vi "DPT Global Test Variables.vi"() -> ()   [LabVIEW 2016, in "File Setup.lvlib"]
uses:
  File Setup.lvlib
  Type Definition/DPT Global Type.ctl
panel:
  in  "34970 RDB Chan":string="101"
  in  "34970 ChTemp Chan":string="113"
  in  "34970 RH Chan":string="112"
  in  "34970 Weight Chan":string="111"
  in  "34970 Label List":string[](array[string])=["RDB F", "Room Ambient(F)", "TC 103", "TC 104", "TC 105", "TC 106", "TC 107", "TC 108", "TC 109", "TC 110"]
  in  "34970 TC Chan List":string="101,102,103,104,105,106,107,108,109,110"
  in  "Corrected Weight Header":string="Corrected Weight"
  in  "Raw Weight Header":string="Raw Weight"
  in  "Weight Header":string="Weight"
  in  "TT3 Header":string="TIME TO 3% RMC:"
  in  "TT4 Header":string="TIME TO 4% RMC:"
  in  "TT5 Header":string="TIME TO 5% RMC:"
  in  "Gas Press Header":string="Gas Pressure"
  in  "Gas Temp Header":string="Gas Temperature"
  in  "Gas Vol Header":string="Gas Feedback"
  in  "Bar. Pressure Header":string="Barometric Pressure"
  in  "WattHour Header":string="Wp:Sigma"
  in  "RMC Header":string="RMC"
  in  "Time Header":string="Time"
  in  "Frequency Label":string="FREQUENCY (Hz):"
  in  "Date Label":string="DATE:"
  in  "IL2 Header":string="Irms:Element 2"
  in  "Dryer On Min Current":dbl=1.0
  in  "IL1 Header":string="Irms:Element 1"
  in  "RH Header":string="Chamber RH"
  in  "Tambient Header":string="Room Ambient(F)"
  in  "VL2 Header":string="Urms:Element 2"
  in  "VL1 Header":string="Urms:Element 1"
  in  "Header Search Key2":string="Date"
  in  "Header Search Key1":string="Time"
  in  "Globals for Dryer Performance Test":T1={"Test Setup"={"RH Resistor"=100.0, "Temp Cal"=72.0, "Temp Coeff"=-0.0234, "Power On Threshold"=50.0, "MA Filter Size"=60, "Weight Offset"=0.0, "Temp Resistor"=100.0, "Gas Enabled"=FALSE, "Gas P. Resistor"=250.0, "Scale Com"=1.0, "W. Samps"=5, "Temp4mA Val"=32.0, "Temp20mA Val"=212.0, "RH4mA Val"=0.0, "RH20mA Val"=100.0, "GPres4mA Val"=0.0, "Gpres20mA Val"=50.0, "Smoothing"=FALSE, "CDAQ"=FALSE, "34970"=FALSE, "34980"=FALSE, "RH-IP"="192.168.1.161", "RH-IP2"="192.168.1.41", "RH-IP3"="192.168.1.42", "CompVolume"=0.0, "T45_Coeff."=0.0}, "Agilent Setup"={"Scale Channel"="3009", "TC Channels"="1001:1040,2001:2040", "VDC Discrete Channels"="3001:3008", "RH Chan"="3010", "Temp Chan"="3011", "Tscale Channel"="1003", "RDB Channel"="1001", "Gas Temperature"="1019", "Gas Pressure"="1020", "Barometric Pressure"="1040", "Gas Feedback Chan"="3012"}, "Directories"={"Work File Directory"=path "c:/Work", "Save File Directory"=path "c:/Data", "Library Directory"=path "c:/Data", "Data Backup Directory"=path "c:/Data", "Data Backup Dir Fail"=path "c:/Data", "Lab Directory"=path "c:/Data"}, "Test Information"={"Model:"="", "Temperature:"="70", "Engineer:"="", "Technician:"="", "Comments:"="", "Lab ID:"="", "TR Number:"="T000000", "Test Number:"="T000000", "Test Station:"="Unitialized", "Empty Dryer Cold Weight:"=0.0, "Serial Number:"="", "Build:"="", "Dryer Type"="", "Humidity"="50", "Test Title per TR:"="Dryer Performance Test"}, "cDAQ Array Locations"={"Scale Channel"="90", "TC Channels"="0-17\n18-35\n36-53\n54-71", "VDC Discrete Channel"="72", "RH Chan"="91", "Temp Chan"="93", "Tscale Channel"="2", "RDB Channel"="0", "Gas Temperature"="88", "Gas Pressure"="89", "Barometric Pressure"="94", "Gas Feedback Chan"="92"}}
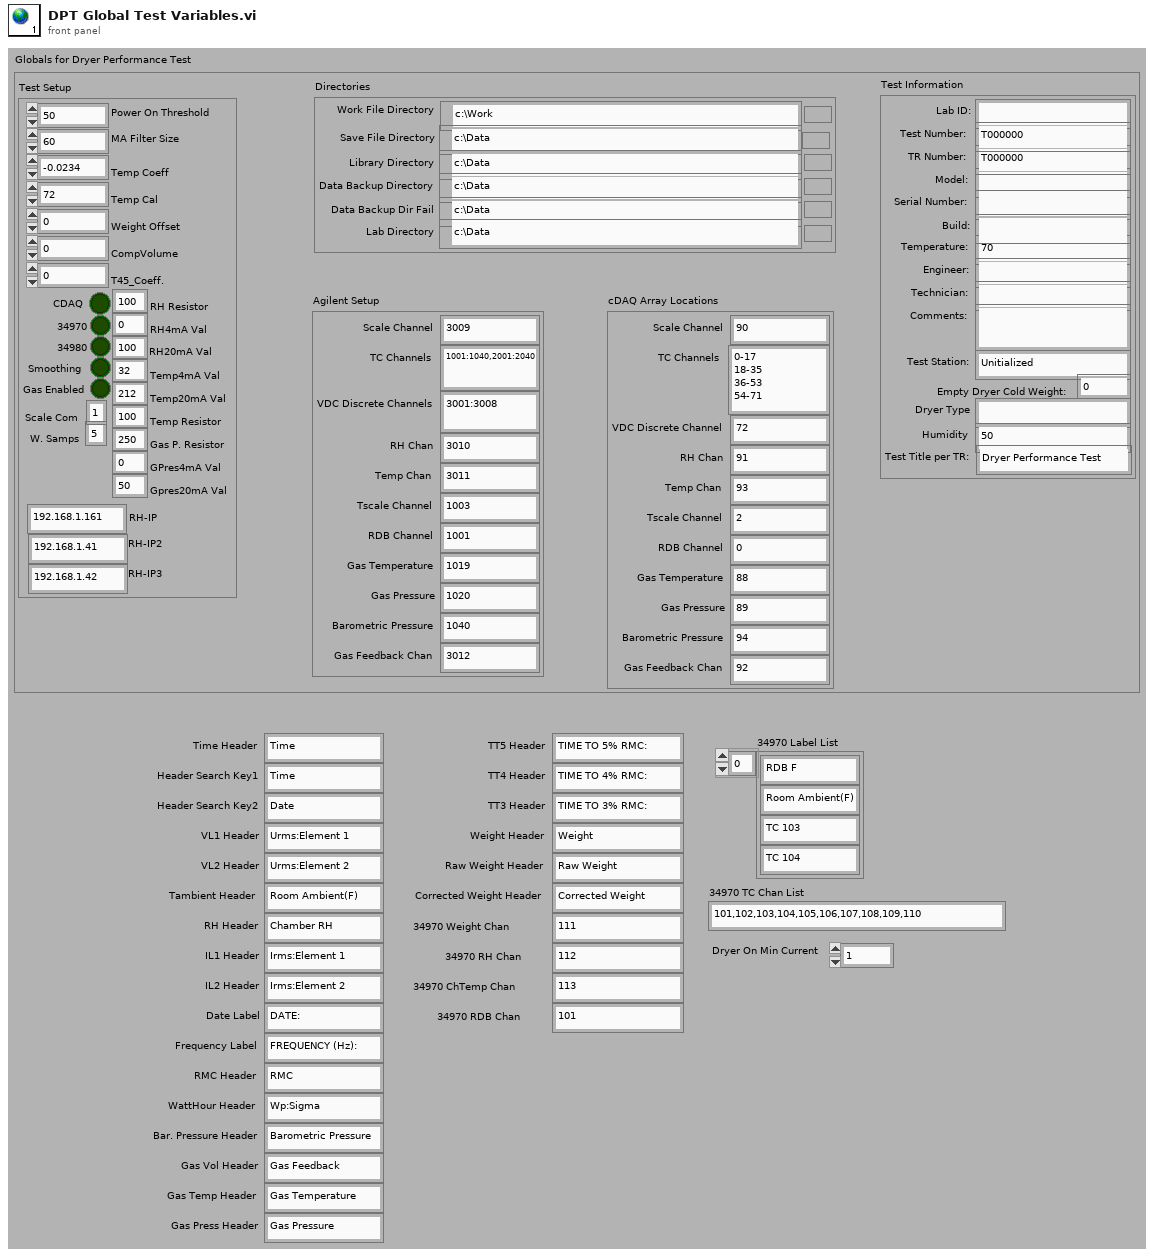
[diagram p1: front panel]
types:
  T1 = typedef "File Setup.lvlib/DPT Global Type.ctl" = cluster{"Test Setup":cluster{"RH Resistor":dbl, "Temp Cal":dbl, "Temp Coeff":dbl, "Power On Threshold":dbl, "MA Filter Size":i32, "Weight Offset":dbl, "Temp Resistor":dbl, "Gas Enabled":bool, "Gas P. Resistor":dbl, "Scale Com":dbl, "W. Samps":i32, "Temp4mA Val":dbl, "Temp20mA Val":dbl, "RH4mA Val":dbl, "RH20mA Val":dbl, "GPres4mA Val":dbl, "Gpres20mA Val":dbl, "Smoothing":bool, "CDAQ":bool, "34970":bool, "34980":bool, "RH-IP":string, "RH-IP2":string, "RH-IP3":string, "CompVolume":dbl, "T45_Coeff.":dbl}, "Agilent Setup":cluster{"Scale Channel":string, "TC Channels":string, "VDC Discrete Channels":string, "RH Chan":string, "Temp Chan":string, "Tscale Channel":string, "RDB Channel":string, "Gas Temperature":string, "Gas Pressure":string, "Barometric Pressure":string, "Gas Feedback Chan":string}, "Directories":cluster{"Work File Directory":path, "Save File Directory":path, "Library Directory":path, "Data Backup Directory":path, "Data Backup Dir Fail":path, "Lab Directory":path}, "Test Information":cluster{"Model:":string, "Temperature:":string, "Engineer:":string, "Technician:":string, "Comments:":string, "Lab ID:":string, "TR Number:":string, "Test Number:":string, "Test Station:":string, "Empty Dryer Cold Weight:":dbl, "Serial Number:":string, "Build:":string, "Dryer Type":string, "Humidity":string, "Test Title per TR:":string}, "cDAQ Array Locations":cluster{"Scale Channel":string, "TC Channels":string, "VDC Discrete Channel":string, "RH Chan":string, "Temp Chan":string, "Tscale Channel":string, "RDB Channel":string, "Gas Temperature":string, "Gas Pressure":string, "Barometric Pressure":string, "Gas Feedback Chan":string}}
diagram:
